vi "Set all gate delays and widths.vi"(6 "Gate B Delay (def: 0 s)":dbl[unit], 7 "Gate A Width (def: 0 s)":dbl[unit], 8 "error in (no error)":errorcluster, 9 "Gate B Width (def: 0 s)":dbl[unit], 10 "Gate A Delay (def: 0 s)":dbl[unit], 11 "VISA resource name":refnum<visa-resource-name>) -> (0 "error out":errorcluster, 3 "VISA resource name out":refnum<visa-resource-name>)   [LabVIEW 2015, in "SR400.lvlib"]
uses:
  SR400.lvlib
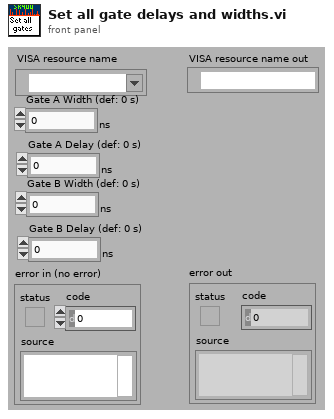
[diagram p1: front panel]
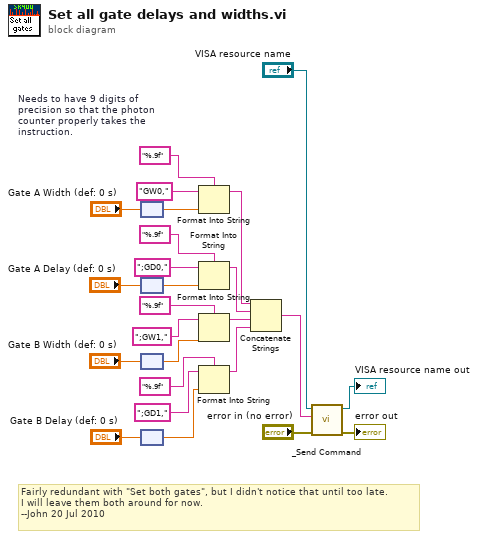
[diagram p0: block diagram]
diagram:
  w24 = "%.9f"  # Needs to have 9 digits of precision so that the photon counter properly takes the instruction.
  # "Fairly redundant with \"Set both gates\", but I didn't notice that until too late.\nI will leave them both around for now.\n--John 20 Jul 2010"
  n1 = node("Gate A Width (def: 0 s)") -> (w7:dbl)
  n2 = node("Gate A Delay (def: 0 s)") -> (w5:dbl)
  n3 = node("Gate B Width (def: 0 s)") -> (w3:dbl)
  n4 = node("Gate B Delay (def: 0 s)") -> (w1:dbl)
  n5 = Format Into String(format string=w24, initial string="GW0," ("command"), w7) -> (resulting string=w17:string)  [unwired: 1 in, 1 out]
  n6 = Format Into String(format string="%.9f" ("Needs to have 9 digits of\nprecision so that the photon\ncounter properly takes the\ninstruction."), initial string=";GD0," ("command"), w5) -> (resulting string=w16:string)  [unwired: 1 in, 1 out]
  n7 = Format Into String(format string="%.9f" ("Needs to have 9 digits of\nprecision so that the photon\ncounter properly takes the\ninstruction."), initial string=";GW1," ("command"), w3) -> (resulting string=w15:string)  [unwired: 1 in, 1 out]
  n8 = Format Into String(format string="%.9f" ("Needs to have 9 digits of\nprecision so that the photon\ncounter properly takes the\ninstruction."), initial string=";GD1," ("command"), w1) -> (resulting string=w14:string)  [unwired: 1 in, 1 out]
  n9 = Concatenate Strings(w17, w16, w15, w14) -> (w10:string)
  n10 = call "_Send Command.vi"("error in (no error)"="error in (no error)", "Command"=w10, "VISA resource name"="VISA resource name") -> ("error out"=→"error out":errorcluster, "VISA resource name out"=→"VISA resource name out":refnum<visa-resource-name>)  [unwired: 1 in, 6 out]
